vi "Write Camera Status.vi"(8 "error in (no error)":errorcluster, 10 "Camera Status":T1, 11 "Camera in":refnum<class "Camera.lvclass">) -> (0 "error out":errorcluster, 3 "Camera out":refnum<class "Camera.lvclass">)   [LabVIEW 2018, in "Camera.lvclass"]
uses:
  Camera.lvclass
  Camera.lvclass/Camera.ctl
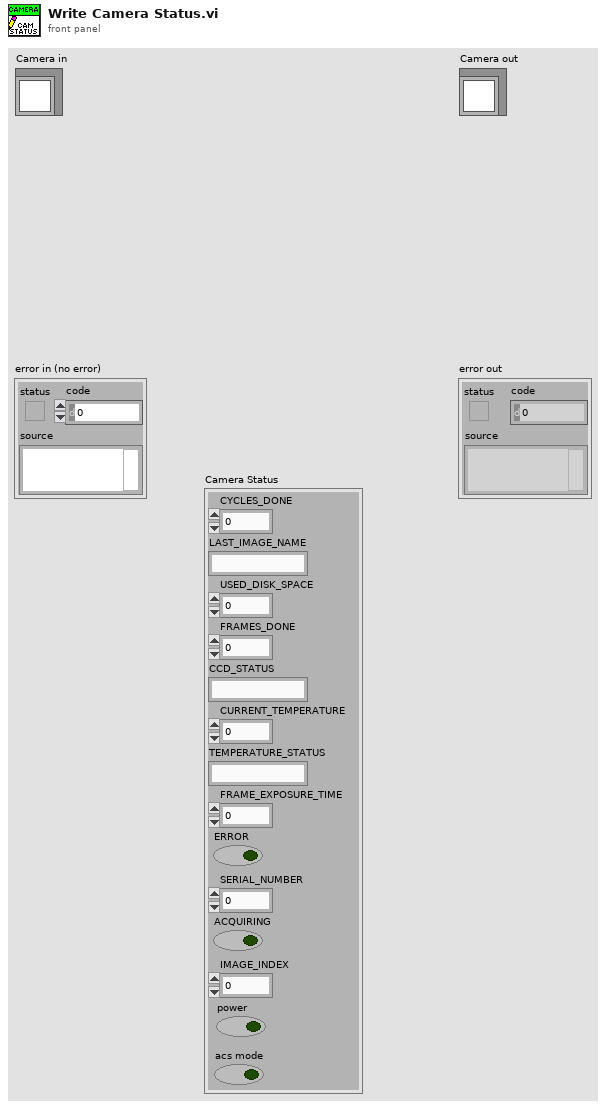
[diagram p1: front panel]
types:
  T1 = cluster{"CYCLES_DONE":u16, "LAST_IMAGE_NAME":string, "USED_DISK_SPACE":u16, "FRAMES_DONE":u16, "CCD_STATUS":string, "CURRENT_TEMPERATURE":i16, "TEMPERATURE_STATUS":string, "FRAME_EXPOSURE_TIME":sgl, "ERROR":bool, "SERIAL_NUMBER":u16, "ACQUIRING":bool, "IMAGE_INDEX":u32, "power":bool, "acs mode":bool}
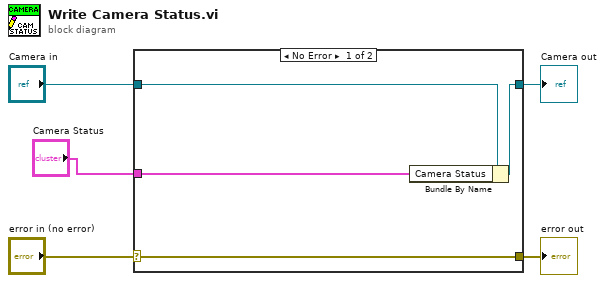
[diagram p0: block diagram]
diagram:
  n1 = case shown="No Error" "error in (no error)" {
    selector: "error in (no error)" -> [w9 w10]
    tunnel: [w9 w10] -> w4
    tunnel: [w7 w11] -> w2
    tunnel: "Camera in" -> [w8 w11]
    tunnel: "Camera Status" -> [w6 _]
    frame No Error {
      n2 = Bundle By Name(cluster=w8, "Camera Status"=w6) -> (w7:refnum<class "Camera.lvclass">)
    }
    frame Error {
    }
  }
  "error out" <- w4
  "Camera out" <- w2
